vi "PT3_Test.vi"() -> ()   [LabVIEW 8.6]
panel:
  out "Stop After (ms)":i32
  out "Stop Reason":enum16{"timeover", "manual", "overflow"}(ring)
  out "Num Records":i32
  out "Header":T1
  out "error out":errorcluster
  in  "error in":errorcluster
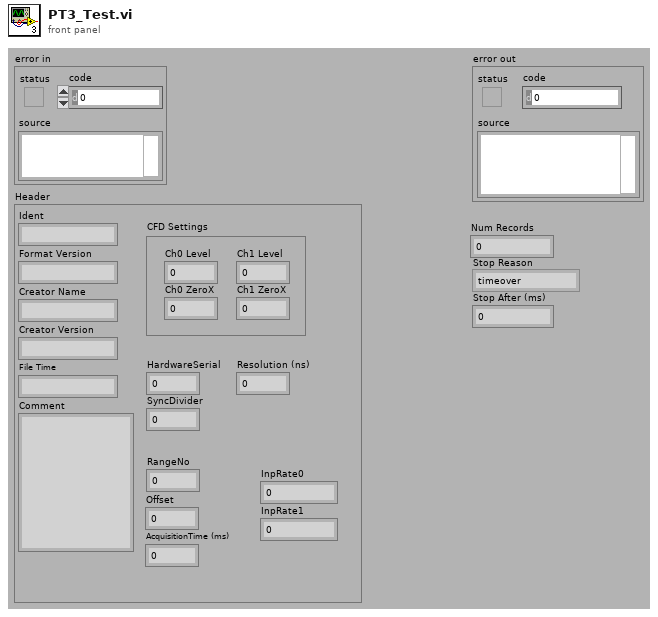
[diagram p1: front panel]
types:
  T1 = cluster{"Ident":string, "Format Version":string, "Creator Name":string, "Creator Version":string, "File Time":string, "Comment":string, "RangeNo":i32, "Offset":i32, "AcquisitionTime (ms)":i32, "HardwareSerial":i32, "SyncDivider":i32, "Resolution (ns)":sgl, "CFD Settings":cluster{"Ch0 Level":i32, "Ch0 ZeroX":i32, "Ch1 Level":i32, "Ch1 ZeroX":i32}, "InpRate0":i32, "InpRate1":i32}
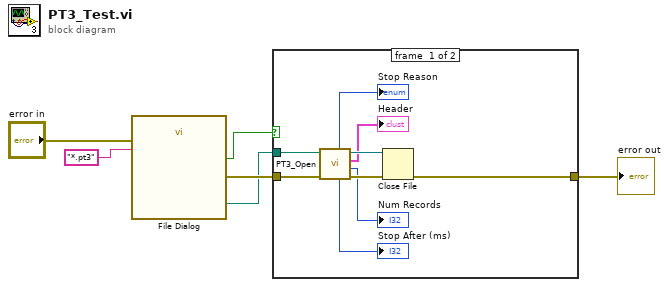
[diagram p0: block diagram]
diagram:
  n1 = call "File Dialog"("error in"="error in", "pattern (all files)"="*.pt3") -> ("selected path"=w4:path, "cancelled"=w3:bool, "error out"=w5:errorcluster)  [unwired: 5 in, 6 out]
  n2 = case shown="False" w3 {
    tunnel: w5 -> [w15 w16]
    tunnel: w4 -> [w14 _]
    tunnel: [w11 w16] -> w2
    frame #0 {
      n3 = call "PT3_Open.vi"("error in"=w15, "File Path"=w14) -> ("error out"=w12:errorcluster, "Num Records"=→"Num Records":i32, "Header"=→"Header":T1, "refnum out"=w13:refnum<file>, "Stop After (ms)"=→"Stop After (ms)":i32, "Stop Reason"=→"Stop Reason":enum16{"timeover", "manual", "overflow"})  [unwired: 4 out]
      n4 = Close File(refnum=w13, error in=w12) -> (error out=w11:errorcluster)  [unwired: 1 out]
    }
    frame #1 {
    }
  }
  "error out" <- w2
